vi "Read Class Type.vi"(8 "error in (no error)":errorcluster, 11 "Domain.lvclass in":refnum<class "NI_Domain.lvclass">) -> (0 "error out":errorcluster, 2 "domain class type":T1 items=["Domain"=0, "Domain_Steady"=100, "Domain_Steady_2D_Rect"=121, "Domain_Steady_2D_Polygon"=122, "Domain_Evolut"=200, "Domain_Evolut_1D"=210, "Domain_Evolut_2D_Rect"=221], 3 "Domain.lvclass out":refnum<class "NI_Domain.lvclass">)   [LabVIEW 2017, in "NI_PDE.lvlib" / "NI_Domain.lvclass"]
uses:
  <vilib>/gmath/pde.llb/DomainClass/NI_Domain.lvclass
  <vilib>/gmath/pde.llb/DomainClass/Class Type.ctl
  <vilib>/gmath/pde.llb/DomainClass/NI_Domain.lvclass/NI_Domain.ctl
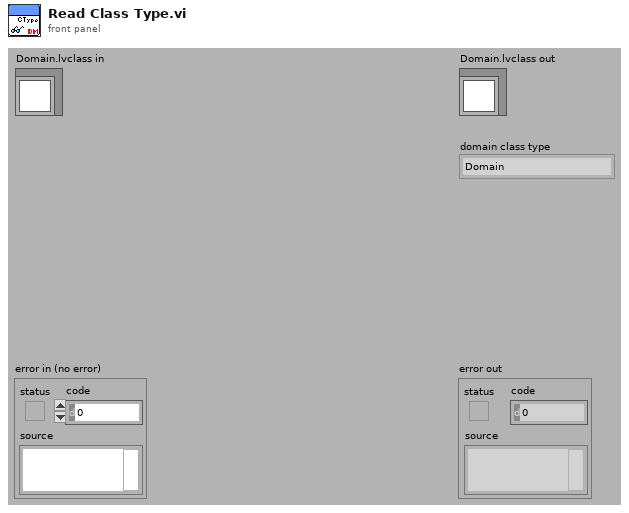
[diagram p1: front panel]
types:
  T1 = typedef "NI_PDE.lvlib/NI_Domain.lvclass/Class Type.ctl" = i32
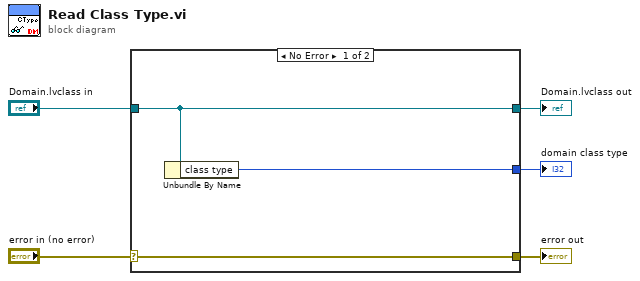
[diagram p0: block diagram]
diagram:
  n1 = case shown="No Error" "error in (no error)" {
    selector: "error in (no error)" -> [w8 w9]
    tunnel: [w8 w9] -> w4
    tunnel: [w7 w10] -> w2
    tunnel: "Domain.lvclass in" -> [w7 w10]
    tunnel: [w6 _] -> w1
    frame No Error {
      n2 = Unbundle By Name(w7) -> ("class type"=w6:T1)
    }
    frame Error {
    }
  }
  "error out" <- w4
  "Domain.lvclass out" <- w2
  "domain class type" <- w1
